vi "GetInformationAboutDb.vi"() -> ()   [LabVIEW 2019]
uses:
  <vilib>/addons/database/Auxilliary.llb/DB Tools DataTypes.ctl
  <vilib>/addons/database/Connection.llb/DB Tools Open Connec (String).vi
  <vilib>/addons/database/NI_Database_API.lvlib
panel:
  out "columns":string[](array[string])
  out "column information":T2(array[cluster])
  out "tables":string[](array[string])
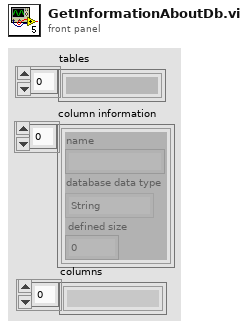
[diagram p1: front panel]
types:
  T1 = typedef "NI_Database_API.lvlib/DB Tools DataTypes.ctl" = enum16{"String", "Long (I32)", "Single (SGL)", "Double (DBL)", "Date/Time", "Binary"}
  T2 = cluster{"name":string, "database data type":T1, "defined size":i32}[]
  T3 = typedef "NI_Database_API.lvlib/Conn ObjectReference.ctl" = refnum<k1>
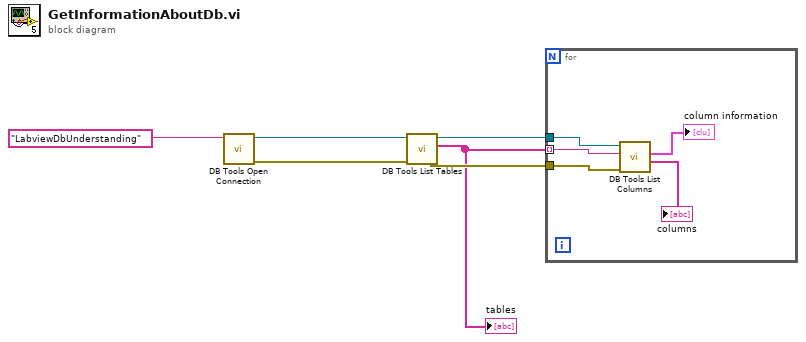
[diagram p0: block diagram]
diagram:
  n1 = call-poly <vilib>:"DB Tools Open Connection.vi"("connection information"="LabviewDbUnderstanding") -> ("error out"=w5:errorcluster, "connection reference"=w6:T3)  [unwired: 7 in]
  n2 = call <vilib>:"DB Tools List Tables.vi"("error in (no error)"=w5, "connection reference"=w6) -> ("error out"=w4:errorcluster, "tables"=w2:string[], "connection reference out"=w3:T3)  [unwired: 3 in]
  "tables" <- w2
  n3 = for {
    tunnel: w4 -> [w11]
    tunnel: w3 -> [w10]
    tunnel: w2 -> [w9] mode=indexing
    n4 = call <vilib>:"DB Tools List Columns.vi"("error in (no error)"=w11, "table"=w9, "connection reference"=w10) -> ("columns"=→"columns":string[], "column information"=→"column information":T2)  [unwired: 1 in, 2 out]
  }
